vi "GetMNValues.vi"(8 "error in (no error)":errorcluster, 10 "Threshold limits":refnum<vi>, 11 "Input ListBox Cluster in":T3) -> (0 "error out":errorcluster, 1 "M and N Array unchanged":T1(array[cluster]), 2 "Input Data Cluster.Rack Selection":T2, 3 "MN Array changed":T1(array[cluster]), 5 "Last ticked measurement":u32)   [LabVIEW 2019, in "ZenGage v3.0 UI.lvclass"]
uses:
  ZenGage v3.0 UI.lvclass
  Type Definitions/Edit tolerance settings/Rack Selection.ctl
  Type Definitions/Edit tolerance settings/Edit Tolerance Input.ctl
  <vilib>/Utility/miscctls.llb/LVPoint32TypeDef.ctl
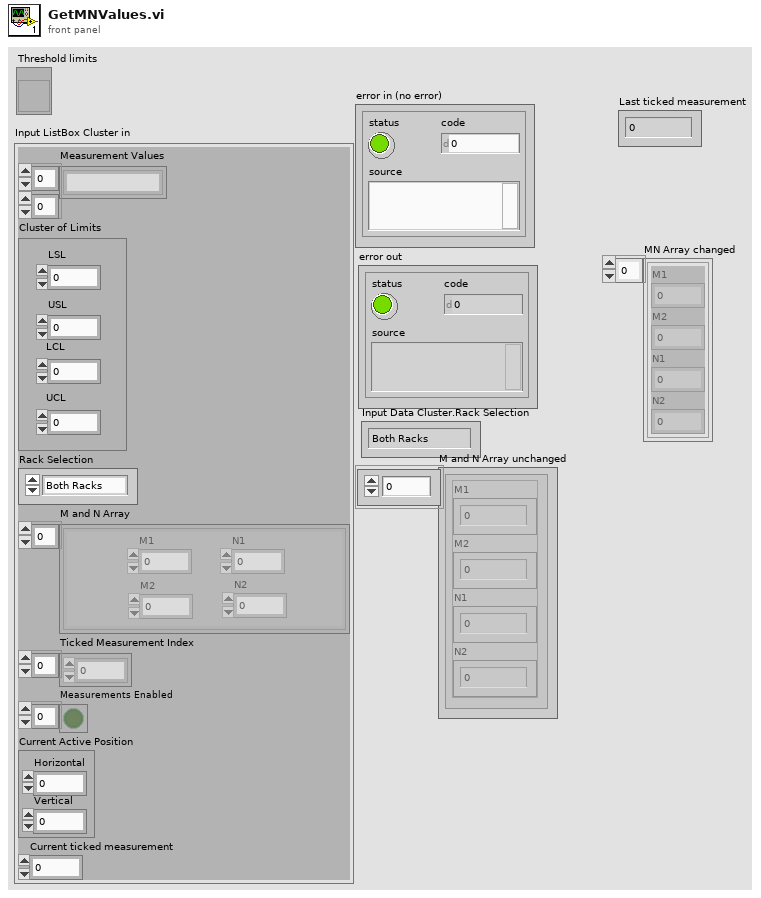
[diagram p1: front panel]
types:
  T1 = cluster{"M1":u64, "M2":u64, "N1":u64, "N2":u64}[]
  T2 = typedef "ZenGage v3.0 UI.lvclass/Rack Selection.ctl" = enum16{"Both Racks", "Rack 2", "Rack 1"}
  T3 = typedef "ZenGage v3.0 UI.lvclass/Edit Tolerance Input.ctl" = cluster{"Measurement Values":string[][], "Cluster of Limits":cluster{"LSL":dbl, "USL":dbl, "LCL":dbl, "UCL":dbl}, "Rack Selection":T2, "M and N Array":cluster{"M1":u64, "M2":u64, "N1":u64, "N2":u64}[], "Ticked Measurement Index":u32[], "Measurements Enabled":bool[], "Current Active Position":T4, "Current ticked measurement":dbl}
  T4 = typedef "LVPoint32TypeDef.ctl" = cluster{"Horizontal":i32, "Vertical":i32}
  T5 = cluster{"Control Limit Fail Allowable":u64, "Spec Limit Fail Allowable":u64, "Control Limit Fail Window":u64, "Spec Limit Fail Window":u64}
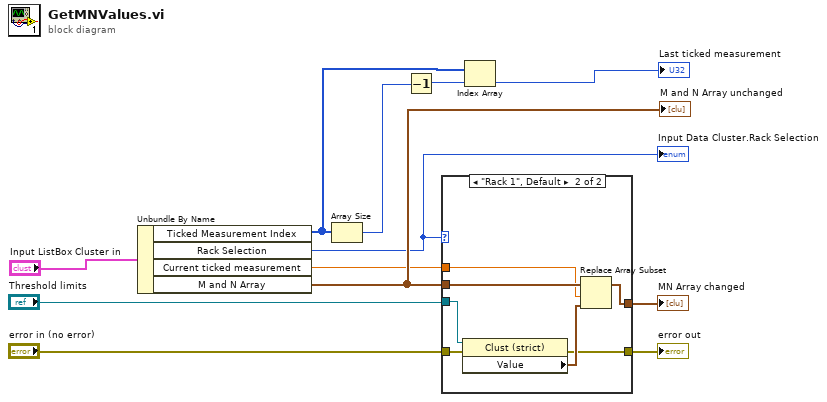
[diagram p0: block diagram]
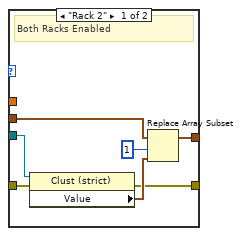
[diagram p2: hidden frame]
diagram:
  n1 = Unbundle By Name("Input ListBox Cluster in") -> ("Ticked Measurement Index"=w2:u32[], "Rack Selection"=w6:T2, "Current ticked measurement"=w7:dbl, "M and N Array"=w8:T1)
  "Input Data Cluster.Rack Selection" <- w6
  "M and N Array unchanged" <- w8
  n2 = Array Size(array=w2) -> (size(s)=w4:i32)
  n3 = Decrement(x=w4) -> (x-1=w3:i32)
  n4 = case shown="\"Rack 1\", Default" w6 {
    tunnel: [w19 w26] -> w12
    tunnel: "Threshold limits" -> [w17 w24]
    tunnel: "error in (no error)" -> [w16 w23]
    tunnel: [w15 w22] -> w9
    tunnel: w8 -> [w14 w21]
    tunnel: w7 -> [_ w20]
    frame "Rack 2" {
      # "Both Racks Enabled"
      n5 = property class="Clust (strict)"(reference=w17, error in=w16) -> (error out=w15:errorcluster, "Value"=w18:T5)  [unwired: 1 out]
      n6 = Replace Array Subset(array=w14, new element=w18, index=1) -> (w19:T1)
    }
    frame "Rack 1", Default {
      n7 = property class="Clust (strict)"(reference=w24, error in=w23) -> (error out=w22:errorcluster, "Value"=w25:T5)  [unwired: 1 out]
      n8 = Replace Array Subset(array=w21, new element=w25, index=w20) -> (w26:T1)
    }
  }
  "MN Array changed" <- w12
  "error out" <- w9
  n9 = Index Array(array=w2, index=w3) -> (element=→"Last ticked measurement":u32)
